vi "GetReportSettings_Mutation.vi"(0 "Diagram":refnum<vi>, 5 "ObjRef":refnum<vi>, 6 "Kind":string="SubVI", 7 "Information":string="<Not A Path>") -> (3 "Replace?":bool)   [LabVIEW 2020]
uses:
  <vilib>/Utility/miscctls.llb/LVPositionTypeDef.ctl
  <vilib>/Utility/Data Type/NI_Data Type.lvlib
  <vilib>/Utility/Data Type/Type Definitions/Data Type.ctl
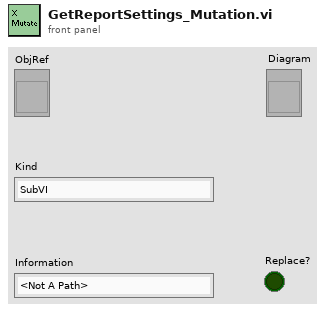
[diagram p1: front panel]
types:
  T1 = typedef "NI_Data Type.lvlib/Data Type.ctl" = enum8{"Invalid Type", "Void", "I8", "I16", "I32", "I64", "U8", "U16", "U32", "U64", "Single Float", "Double Float", "Extended Float", "Single Complex", "Double Complex", "Extended Complex", "Enum U8", "Enum U16", "Enum U32", "Enum U64", "Single Float With Unit", "Double Float With Unit", "Extended Float With Unit", "Single Complex with Unit", "Double Complex with Unit", "Extended Complex with Unit", "Boolean", "String", "Path", "Picture", "Tag", "Array", "Cluster", "Variant", "LV Variant", "Waveform", "Timestamp", "Digital Waveform", "Digital Data", "ExpressData", "Refnum", "External Data", "VI", "Poly VI", "LabVIEW Class Instance", "Fixed Point", "Set Collection", "Map Collection"}
  T2 = typedef "LVPositionTypeDef.ctl" = cluster{"Left":i32, "Top":i32}
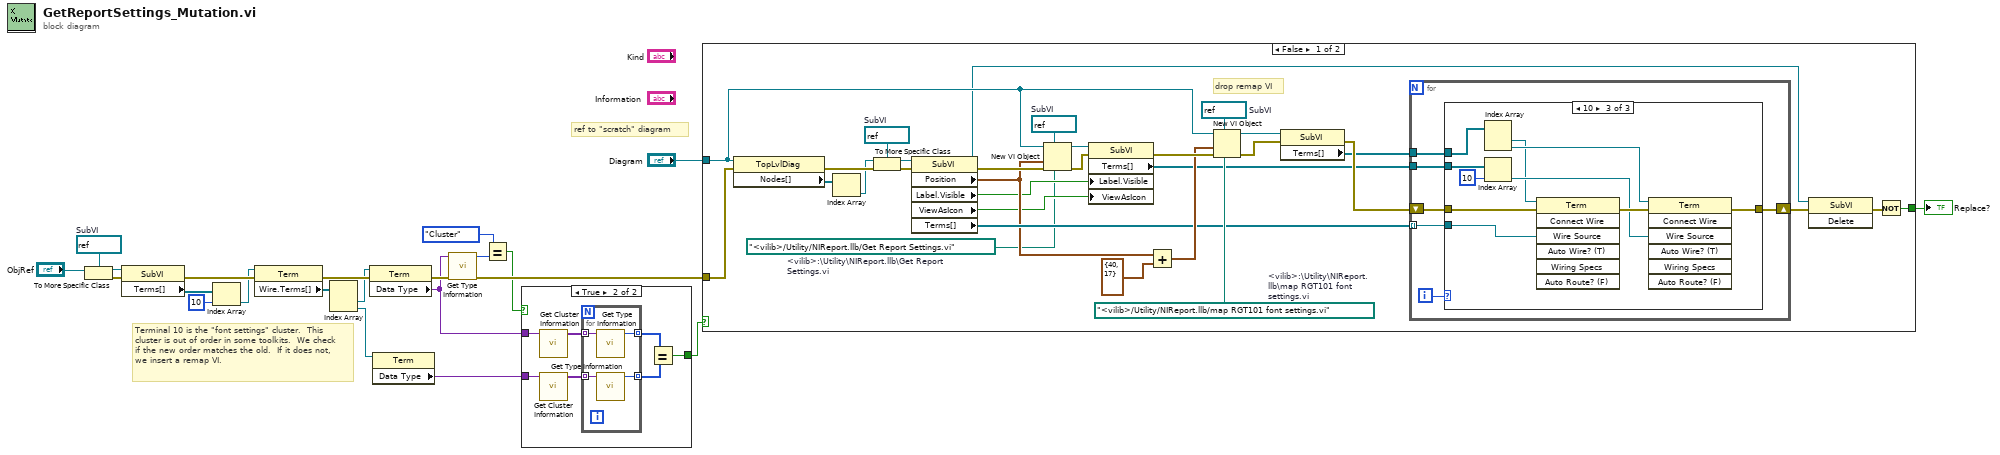
[diagram p0: block diagram]
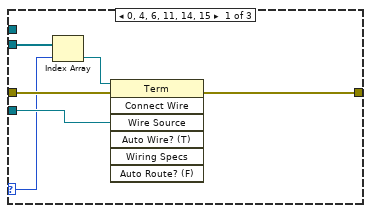
[diagram p2: hidden frame]
diagram:
  w15 = refnum<vi> refnum  # SubVI
  # "Terminal 10 is the \"font settings\" cluster.  This cluster is out of order in some toolkits.  We check if the new order matches the old.  If it does not, we insert a remap VI."
  # "ref to \"scratch\" diagram"
  n1 = To More Specific Class(target class=w15, reference="ObjRef") -> (specific class reference=w13:refnum<vi>, error out=w22:errorcluster)  [unwired: 1 in]
  n2 = property class="SubVI"(reference=w13, error in=w22) -> (error out=w21:errorcluster, "Terms[]"=w12:refnum<vi>[])  [unwired: 1 out]
  n3 = Index Array(array=w12, index=10) -> (element=w10:refnum<vi>)
  n4 = property class="Term"(reference=w10, error in=w21) -> (error out=w20:errorcluster, "Wire.Terms[]"=w9:refnum<vi>[])  [unwired: 1 out]
  n5 = Index Array(array=w9) -> (element #1=w8:refnum<vi>, element #2=w5:refnum<vi>)  [unwired: 2 in]
  n6 = property class="Term"(reference=w8, error in=w20) -> (error out=w19:errorcluster, "Data Type"=w6:variant)  [unwired: 1 out]
  n7 = property class="Term"(reference=w5) -> ("Data Type"=w4:variant)  [unwired: 1 in, 2 out]
  n8 = call <vilib>:"Get Type Information.vi"("error in (no error)"=w19, "variant"=w6) -> ("error out"=w18:errorcluster, "type"=w7:T1)  [unwired: 5 in, 3 out]
  n9 = Equal?(x=Data_Type."Cluster", y=w7) -> (x = y?=w3:bool)
  n10 = case shown="True" w3 {
    tunnel: w6 -> [_ w29]
    tunnel: w4 -> [_ w28]
    tunnel: [_ w23] -> w2
    frame False {
    }
    frame True {
      n11 = call <vilib>:"Get Cluster Information.vi"("variant"=w29) -> ("cluster elements"=w27:variant[])  [unwired: 9 in, 1 out]
      n12 = call <vilib>:"Get Cluster Information.vi"("variant"=w28) -> ("cluster elements"=w26:variant[])  [unwired: 9 in, 1 out]
      n13 = for {
        tunnel: w27 -> [w33] mode=indexing
        tunnel: w26 -> [w32] mode=indexing
        tunnel: [w31] -> w25 mode=indexing
        tunnel: [w30] -> w24 mode=indexing
        n14 = call <vilib>:"Get Type Information.vi"("variant"=w33) -> ("type"=w31:T1)  [unwired: 6 in, 4 out]
        n15 = call <vilib>:"Get Type Information.vi"("variant"=w32) -> ("type"=w30:T1)  [unwired: 6 in, 4 out]
      }
      n16 = Equal?(x=w25, y=w24) -> (x = y?=w23:bool)
    }
  }
  n17 = case shown="False" w2 {
    tunnel: "Diagram" -> [w41 _]
    tunnel: [w50 _] -> w16
    tunnel: w18 -> [w60 _]
    frame False {
      w35 = path "<vilib>/Utility/NIReport.llb/Get Report Settings.vi"  # <vilib>:\Utility\NIReport.llb\Get Report Settings.vi
      w42 = refnum<vi> refnum  # SubVI
      w46 = path "<vilib>/Utility/NIReport.llb/map RGT101 font settings.vi"  # <vilib>:\Utility\NIReport.llb\map RGT101 font settings.vi
      w49 = refnum<vi> refnum  # SubVI
      w54 = refnum<vi> refnum  # SubVI
      # "drop remap VI"
      n18 = property class="TopLvlDiag"(reference=w41, error in=w60) -> (error out=w64:errorcluster, "Nodes[]"=w53:refnum<vi>[])  [unwired: 1 out]
      n19 = Index Array(array=w53) -> (element=w52:refnum<vi>)  [unwired: 1 in]
      n20 = To More Specific Class(target class=w54, reference=w52, error in=w64) -> (specific class reference=w51:refnum<vi>, error out=w63:errorcluster)
      n21 = property class="SubVI"(reference=w51, error in=w63) -> (reference out=w40:refnum<vi>, error out=w59:errorcluster, "Position"=w38:T2, "Label.Visible"=w37:bool, "ViewAsIcon"=w36:bool, "Terms[]"=w43:refnum<vi>[])
      n22 = New VI Object(vi object class=w42, owner refnum=w41, position/next to=w38, 6:w35, 8:w59) -> (object refnum=w39:refnum<vi>, 0:w56:errorcluster)  [unwired: 3 in]
      n23 = property class="SubVI"(reference=w39, error in=w56, "Label.Visible"=w37, "ViewAsIcon"=w36) -> (error out=w55:errorcluster, "Terms[]"=w34:refnum<vi>[])  [unwired: 1 out]
      n24 = Add(x=w38, y=T2 {"Left"=40, "Top"=17}) -> (x+y=w44:T2)
      n25 = New VI Object(vi object class=w49, owner refnum=w41, position/next to=w44, 6:w46, 8:w55) -> (object refnum=w47:refnum<vi>, 0:w62:errorcluster)  [unwired: 3 in]
      n26 = property class="SubVI"(reference=w47, error in=w62) -> (error out=w61:errorcluster, "Terms[]"=w48:refnum<vi>[])  [unwired: 1 out]
      n27 = for {
        tunnel: w43 -> [w67] mode=indexing
        tunnel: w48 -> [w65]
        shift-right: [w69] -> w58
        shift-left: w61 -> [w70]
        tunnel: w34 -> [w66]
        i -> [w68]
        n28 = case shown="10" w68 {
          selector: w68 -> [w71 _ _]
          tunnel: w67 -> [w74 _ w84]
          tunnel: w66 -> [w73 _ w83]
          tunnel: w70 -> [w76 w77 w87]
          tunnel: [w75 w77 w85] -> w69
          tunnel: w65 -> [_ _ w81]
          frame 0, 4, 6, 11, 14, 15 {
            n29 = Index Array(array=w73, index=w71) -> (element=w72:refnum<vi>)
            n30 = invoke class="Term" method="Connect Wire"(reference=w72, error in=w76, "Wire Source"=w74) -> (error out=w75:errorcluster)  [unwired: 4 in, 6 out]
          }
          frame 1..3, 5, 7..9, 12, 13, Default {
          }
          frame 10 {
            n31 = Index Array(array=w81) -> (element #1=w78:refnum<vi>, element #2=w79:refnum<vi>)  [unwired: 2 in]
            n32 = Index Array(array=w83, index=10) -> (element=w80:refnum<vi>)
            n33 = invoke class="Term" method="Connect Wire"(reference=w78, error in=w87, "Wire Source"=w84) -> (error out=w86:errorcluster)  [unwired: 4 in, 6 out]
            n34 = invoke class="Term" method="Connect Wire"(reference=w79, error in=w86, "Wire Source"=w80) -> (error out=w85:errorcluster)  [unwired: 4 in, 6 out]
          }
        }
      }
      n35 = invoke class="SubVI" method="Delete"(reference=w40, error in=w58) -> (error out=w57:errorcluster)  [unwired: 1 in, 2 out]
      n36 = Not(x=w57) -> (.not. x?=w50:bool)
    }
    frame True {
      # "The \"font settings\" cluster is the same on both ends, so do nothing."
    }
  }
  "Replace?" <- w16
